vi "DN4_DI_Read.vi"(0 "Task ID":u32, 1 "error in (no error)":errorcluster) -> (2 "Task ID":u32, 3 "data out":u8[](array[numeric]), 4 "error out":errorcluster)   [LabVIEW 2009]
uses:
  Windows/System32/AdvLvDaq.dll
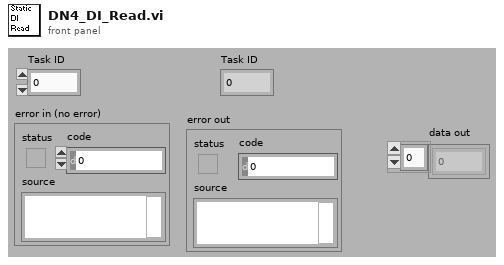
[diagram p1: front panel]
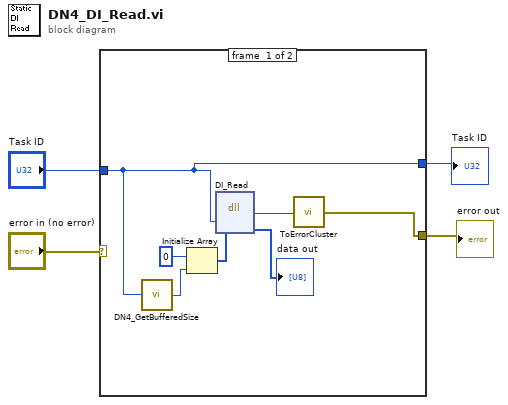
[diagram p0: block diagram]
diagram:
  n1 = case shown="No Error" "error in (no error)" {
    selector: "error in (no error)" -> [_ w12]
    tunnel: "Task ID" -> [w6 w13]
    tunnel: [w10 w12] -> w3
    tunnel: [w6 w13] -> w2
    frame #0 {
      n2 = call <userlib>:"DN4_GetBufferedSize.vi"("Task ID"=w6) -> ("return type"=w7:i32)
      n3 = Initialize Array(u8 0 ("element"), w7) -> (w5:u8[])
      n4 = dll-call lib="C:/Windows/System32/AdvLvDaq.dll" fn="DI_Read"("taskId"=w6, "data"=w5) -> ("return type"=w11:i32, "data"=→"data out":u8[])  [unwired: 4 in, 2 out]
      n5 = call <userlib>:"ToErrorCluster.vi"("error code"=w11) -> ("error out"=w10:errorcluster)
    }
    frame #1 {
    }
  }
  "error out" <- w3
  "Task ID" <- w2
